vi "Create Name Actor.vi"(6 "Name Actor":string, 8 "error in":errorcluster, 9 "Name Library File Path":path, 10 "Active Project":refnum<vi>) -> (0 "error out":errorcluster, 2 "Name Actor":T1)   [LabVIEW 2025, in "_Rescript.lvlib" / "Actor.lvlib" / "Actor.lvclass"]
uses:
  Actor.lvclass
  Actor.lvclass/Actor.ctl
  Attributes.ctl
  _Rescript.lvlib
  Terminal Attributes.ctl
  Name Actor.ctl
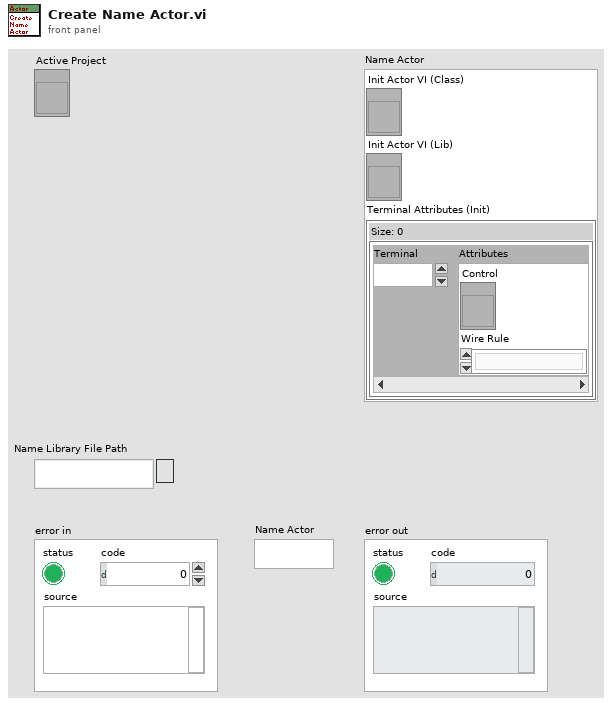
[diagram p1: front panel]
types:
  T1 = typedef "_Rescript.lvlib/Actor.lvlib/Actor.lvclass/Name Actor.ctl" = cluster{"Init Actor VI (Class)":refnum<vi>, "Init Actor VI (Lib)":refnum<vi>, "Terminal Attributes (Init)":T2}
  T2 = typedef "_Rescript.lvlib/Terminal Attributes.ctl" = map{i32, T3}
  T3 = typedef "_Rescript.lvlib/Attributes.ctl" = cluster{"Control":refnum<vi>, "Wire Rule":enum16{"Invalid Wire Rule", "Required", "Recommended", "Optional", "Dynamic Dispatch"}}
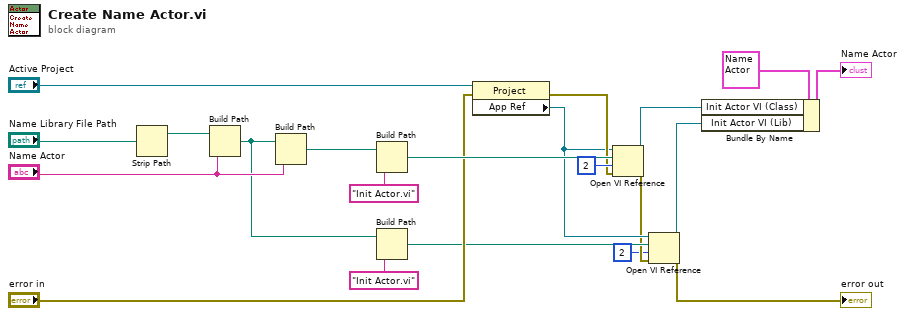
[diagram p0: block diagram]
diagram:
  n1 = Strip Path(path="Name Library File Path") -> (stripped path=w18:path)  [unwired: 1 out]
  n2 = Build Path(base path=w18, name or relative path="Name Actor") -> (appended path=w7:path)
  n3 = Build Path(base path=w7, name or relative path="Name Actor") -> (appended path=w16:path)
  n4 = Build Path(base path=w16, name or relative path="Init Actor.vi" ("format string")) -> (appended path=w20:path)
  n5 = Build Path(base path=w7, name or relative path="Init Actor.vi" ("format string")) -> (appended path=w6:path)
  n6 = property class="Project"(reference="Active Project", error in="error in") -> (error out=w9:errorcluster, "App Ref"=w5:refnum<vi>)  [unwired: 1 out]
  n7 = Open VI Reference(application reference (local)=w5, vi path=w20, options=2, error in (no error)=w9) -> (vi reference=w17:refnum<vi>, error out=w4:errorcluster)  [unwired: 2 in]
  n8 = Open VI Reference(application reference (local)=w5, vi path=w6, options=2, error in (no error)=w4) -> (vi reference=w1:refnum<vi>, error out=→"error out":errorcluster)  [unwired: 2 in]
  n9 = Bundle By Name(cluster=T1 {"Init Actor VI (Class)"=refnum, "Init Actor VI (Lib)"=refnum, "Terminal Attributes (Init)"={}} ("Name Actor"), "Init Actor VI (Class)"=w17, "Init Actor VI (Lib)"=w1) -> (→"Name Actor":T1)
